vi "VI Anlagenuebersicht_PNS.vi"() -> (3 "XML-String":string)   [LabVIEW 2020, in "PNS.lvlib" / "PNS Anlagenuebersicht.lvlib"]
uses:
  PNS Anlagenuebersicht.lvlib
  PNS Ventile.ctl
  Aktionen FGV Grenzwerte.ctl
  PNS.lvlib
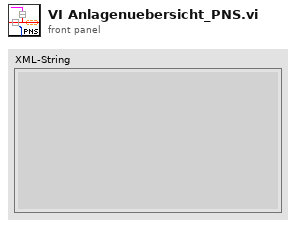
[diagram p1: front panel]
types:
  T1 = typedef "PNS.lvlib/Aktionen FGV Grenzwerte.ctl" = enum16{"lesen", "Grenzw. schreiben", "Anweisungscode", "IP-Adresse", "laden", "speichern", "Anweisungscode vorgeben"}
  T2 = typedef "PNS.lvlib/PNS Anlagenuebersicht.lvlib/PNS Ventile.ctl" = cluster{"-Y01 Spülen ":bool, "-Y02 Lüften ":bool, "-Y03 Cal Gas":bool, "-Y04 Eingang":bool, "-Y05 Messen 01":bool, "-Y06 Messen 02":bool, "-Y07 Messen 03":bool, "-Y08 Messen 04":bool, "-Y09 Messen 05":bool, "-Y10 Messen 06":bool, "-Y11 Messen 07":bool, "-Y12 Messen 08":bool}
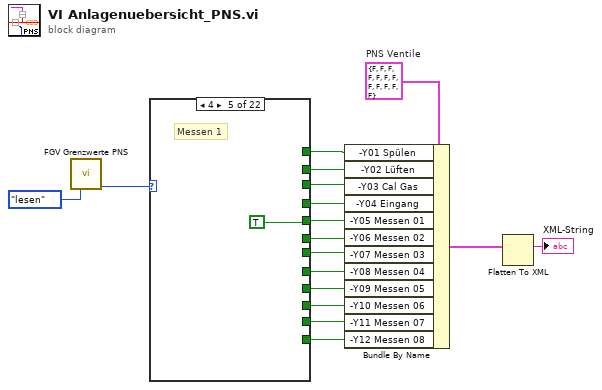
[diagram p0: block diagram]
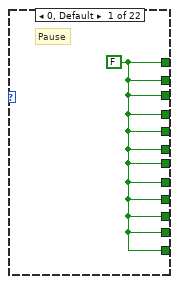
[diagram p2: hidden frame]
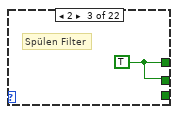
[diagram p4: hidden frame]
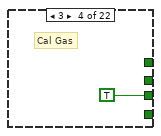
[diagram p5: hidden frame]
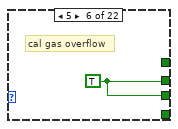
[diagram p6: hidden frame]
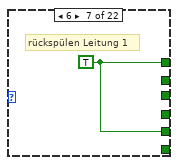
[diagram p7: hidden frame]
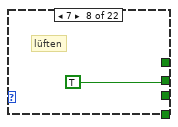
[diagram p8: hidden frame]
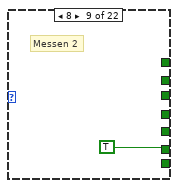
[diagram p9: hidden frame]
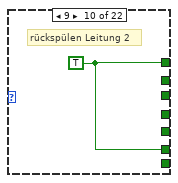
[diagram p10: hidden frame]
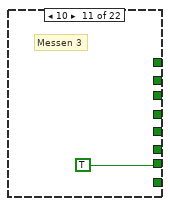
[diagram p11: hidden frame]
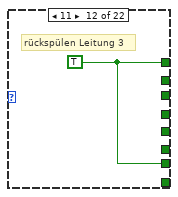
[diagram p12: hidden frame]
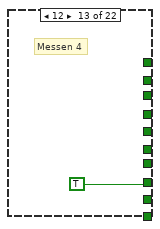
[diagram p13: hidden frame]
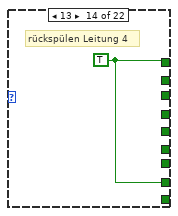
[diagram p14: hidden frame]
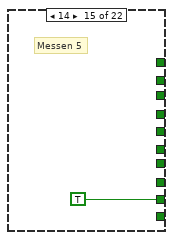
[diagram p15: hidden frame]
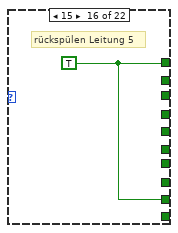
[diagram p16: hidden frame]
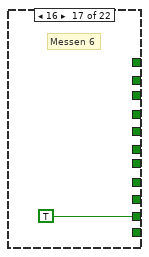
[diagram p17: hidden frame]
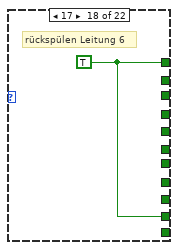
[diagram p18: hidden frame]
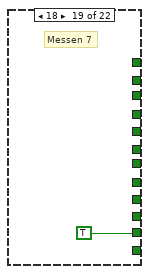
[diagram p19: hidden frame]
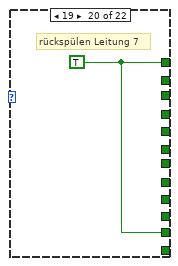
[diagram p20: hidden frame]
diagram:
  w15 = T2 {"-Y01 Spülen "=FALSE, "-Y02 Lüften "=FALSE, "-Y03 Cal Gas"=FALSE, "-Y04 Eingang"=FALSE, "-Y05 Messen 01"=FALSE, "-Y06 Messen 02"=FALSE, "-Y07 Messen 03"=FALSE, "-Y08 Messen 04"=FALSE, "-Y09 Messen 05"=FALSE, "-Y10 Messen 06"=FALSE, "-Y11 Messen 07"=FALSE, "-Y12 Messen 08"=FALSE}  # PNS Ventile
  n1 = call "FGV Grenzwerte PNS.vi"("Aktionen FGV Grenzwerte"=Aktionen_FGV_Grenzwerte."lesen") -> ("Anweisungscode"=w16:u16)  [unwired: 12 in, 2 out]
  n2 = case shown="4" w16 {
    tunnel: [w18 _ w19 _ _ _ w23 _ _ w26 _ w28 _ w30 _ w32 _ w34 _ w36 _ w38] -> w12
    tunnel: [w18 _ w19 _ _ w22 _ TRUE _ _ _ _ _ _ _ _ _ _ _ _ _ _] -> w11
    tunnel: [w18 _ _ TRUE _ w22 _ _ _ _ _ _ _ _ _ _ _ _ _ _ _ _] -> w10
    tunnel: [w18 _ _ _ _ _ _ _ _ _ _ _ _ _ _ _ _ _ _ _ _ _] -> w9
    tunnel: [w18 _ _ _ TRUE _ w23 _ _ _ _ _ _ _ _ _ _ _ _ _ _ _] -> w8
    tunnel: [w18 _ _ _ _ _ _ _ TRUE w26 _ _ _ _ _ _ _ _ _ _ _ _] -> w7
    tunnel: [w18 _ _ _ _ _ _ _ _ _ TRUE w28 _ _ _ _ _ _ _ _ _ _] -> w6
    tunnel: [w18 _ _ _ _ _ _ _ _ _ _ _ TRUE w30 _ _ _ _ _ _ _ _] -> w5
    tunnel: [w18 _ _ _ _ _ _ _ _ _ _ _ _ _ TRUE w32 _ _ _ _ _ _] -> w4
    tunnel: [w18 _ _ _ _ _ _ _ _ _ _ _ _ _ _ _ TRUE w34 _ _ _ _] -> w3
    tunnel: [w18 _ _ _ _ _ _ _ _ _ _ _ _ _ _ _ _ _ TRUE w36 _ _] -> w2
    tunnel: [w18 _ _ _ _ _ _ _ _ _ _ _ _ _ _ _ _ _ _ _ TRUE w38] -> w1
    frame 0, Default {
      w18 = FALSE
      # "Pause"
    }
    frame 1 {
      # "Standby"
    }
    frame 2 {
      w19 = TRUE
      # "Spülen Filter"
    }
    frame 3 {
      # "Cal Gas"
    }
    frame 4 {
      # "Messen 1"
    }
    frame 5 {
      w22 = TRUE
      # "cal gas overflow"
    }
    frame 6 {
      w23 = TRUE
      # "rückspülen Leitung 1"
    }
    frame 7 {
      # "lüften"
    }
    frame 8 {
      # "Messen 2"
    }
    frame 9 {
      w26 = TRUE
      # "rückspülen Leitung 2"
    }
    frame 10 {
      # "Messen 3"
    }
    frame 11 {
      w28 = TRUE
      # "rückspülen Leitung 3"
    }
    frame 12 {
      # "Messen 4"
    }
    frame 13 {
      w30 = TRUE
      # "rückspülen Leitung 4"
    }
    frame 14 {
      # "Messen 5"
    }
    frame 15 {
      w32 = TRUE
      # "rückspülen Leitung 5"
    }
    frame 16 {
      # "Messen 6"
    }
    frame 17 {
      w34 = TRUE
      # "rückspülen Leitung 6"
    }
    frame 18 {
      # "Messen 7"
    }
    frame 19 {
      w36 = TRUE
      # "rückspülen Leitung 7"
    }
    frame 20 {
      # "Messen 8"
    }
    frame 21 {
      w38 = TRUE
      # "rückspülen Leitung 8"
    }
  }
  n3 = Bundle By Name(cluster=w15, "-Y01 Spülen"=w12, "-Y02 Lüften"=w11, "-Y03 Cal Gas"=w10, "-Y04 Eingang"=w9, "-Y05 Messen 01"=w8, "-Y06 Messen 02"=w7, "-Y07 Messen 03"=w6, "-Y08 Messen 04"=w5, "-Y09 Messen 05"=w4, "-Y10 Messen 06"=w3, "-Y11 Messen 07"=w2, "-Y12 Messen 08"=w1) -> (w14:T2)
  n4 = Flatten To XML(6:w14) -> (2:→"XML-String":string)
